vi "P116x2ch_WriteManual.vi"(5 "P116x2":T1, 7 "Enable(T)":bool=TRUE, 8 "error in (no error)":errorcluster, 9 "RateSP":T2, 10 "NuevoSP":T2, 11 "VISA Eurotherm":refnum<visa-resource-name>) -> (0 "error out":errorcluster, 1 "RateSP_out":T2, 2 "NuevoSP_out":T2)   [LabVIEW 2017]
uses:
  2xP116.ctl
  _P2024_P116x2w.ctl
  Address.ctl
  Eurotherm_2023_Module.ctl
  P2024 TB ICB GLOBALES.vi
panel:
  out "PV":T2
  out "WorkingSP":T2
  out "TargetSP":T2
  in  "Cancel":bool
  in  "Write":bool
  in  "Delay Time (s)":dbl=0.1
  # "Programando controladores P116"
  # "C/min"
  # "C"
  # "C"
  # "C"
  # "C"
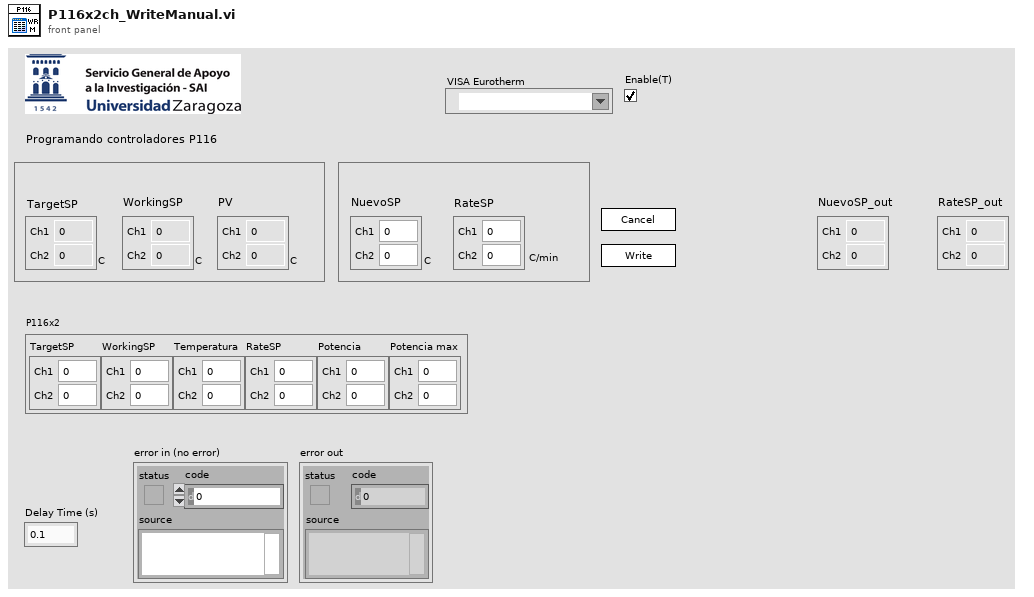
[diagram p1: front panel]
types:
  T1 = typedef "_P2024_P116x2w.ctl" = cluster{"TargetSP":T2, "WorkingSP":T2, "Temperatura":T2, "RateSP":T2, "Potencia":T2, "Potencia max":T2}
  T2 = typedef "2xP116.ctl" = cluster{"Ch1":dbl, "Ch2":dbl}
  T3 = typedef "_P2024 COMMS.ctl" = cluster{"Alicat":refnum<visa-resource-name>, "eAlic":bool, "Eurotherm":refnum<visa-resource-name>, "eEurot":bool, "Balanza":refnum<visa-resource-name>, "eBal":bool, "Valvula":refnum<visa-resource-name>, "eVal":bool}
  T4 = typedef "Eurotherm_2023_Module.ctl" = enum16{"Initialize", "Write setpoint", "Read data", "Write ramp rate", "Set constante proporcional", "Set constante integral", "Set constante diferencial", "Set ouput limit LOW", "Set ouput limit HIGH", "Shutdown"}
  T5 = typedef "Address.ctl" = enum16{"Add 1", "Add 2", "Add 3", "Add 4", "Add 5", "Add 6", "Add 10", "Add 11", "Add 12", "Add 13"}
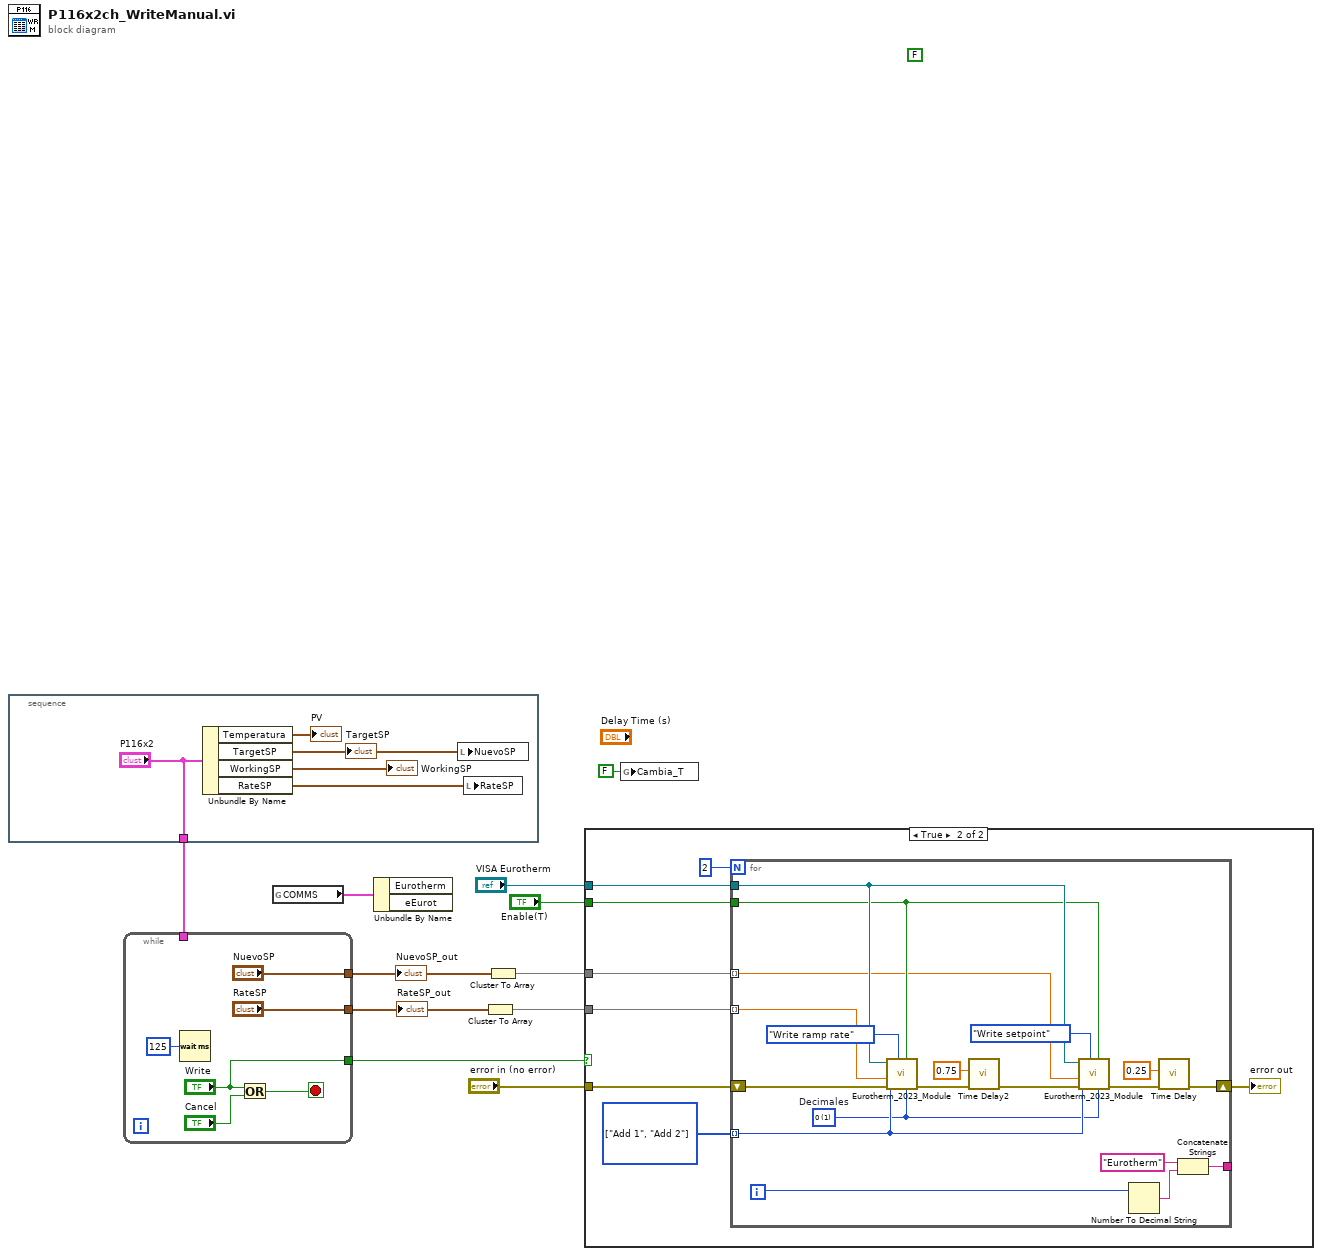
[diagram p0: block diagram]
diagram:
  (unwired) FALSE
  n1 = stacked-sequence {
    tunnel: ["P116x2"] -> w3
    frame #0 {
      n2 = Unbundle By Name("P116x2") -> ("Temperatura"=→"PV":T2, "TargetSP"=w14:T2, "WorkingSP"=→"WorkingSP":T2, "RateSP"=w12:T2)
      "TargetSP" <- w14
      n3 = local write "NuevoSP"(w14) -> ()
      n4 = local write "RateSP"(w12) -> ()
    }
  }
  n5 = while {
    tunnel: ["NuevoSP"] -> w1
    tunnel: ["RateSP"] -> w2
    tunnel: ["Write"] -> w6
    tunnel: w3 -> [_]
    stop <- w17 stop-if-true
    n6 = Wait (ms)(milliseconds to wait=u32 125) -> ()  [unwired: 1 out]
    n7 = Or(x="Write", y="Cancel") -> (x .or. y?=w17:bool)
  }
  "NuevoSP_out" <- w1
  "RateSP_out" <- w2
  n8 = global read "P2024 TB ICB GLOBALES.vi" "COMMS"() -> (w11:T3)
  n9 = Unbundle By Name(w11) -> ()  [unwired: 2 out]
  n10 = Cluster To Array(cluster=w2) -> (array=w7:dbl[])
  n11 = Cluster To Array(cluster=w1) -> (array=w8:dbl[])
  n12 = case shown="True" w6 {
    tunnel: "Enable(T)" -> [_ w29]
    tunnel: "error in (no error)" -> [_ w27]
    tunnel: w8 -> [_ w25]
    tunnel: w7 -> [_ w26]
    tunnel: "VISA Eurotherm" -> [_ w30]
    frame False {
    }
    frame True {
      w23 = T5[] [enum."Add 1", enum."Add 2"] items=["Add 1", "Add 2", "Add 3", "Add 4", "Add 5", "Add 6", "Add 10", "Add 11", "Add 12", "Add 13"]
      n13 = for {
        N: 2 -> [_]
        tunnel: w23 -> [w32] mode=indexing
        shift-right: [w37] -> w28
        shift-left: w27 -> [w44]
        tunnel: [w47] -> _
        tunnel: w25 -> [w39] mode=indexing
        tunnel: w26 -> [w40] mode=indexing
        tunnel: w30 -> [w43]
        tunnel: w29 -> [w42]
        i -> [w36]
        w31 = u16 1 items=["0"=1, "1"=10, "2"=100]  # Decimales
        n14 = call "Eurotherm_2023_Module.vi"("Decimales"=w31, "Eurotherm (T:Enable)"=w42, "Command"=Eurotherm_2023_Module."Write ramp rate", "error in (no error)"=w44, "Value"=w40, "Address"=w32, "VISA resource name"=w43) -> ("error out"=w34:errorcluster)  [unwired: 3 in, 1 out]
        n15 = call "Time Delay2"("error in (no error)"=w34, "Delay Time (s)"=0.75) -> ("error out"=w33:errorcluster)  [unwired: 9 in]
        n16 = call "Eurotherm_2023_Module.vi"("Decimales"=w31, "Eurotherm (T:Enable)"=w42, "Command"=Eurotherm_2023_Module."Write setpoint", "error in (no error)"=w33, "Value"=w39, "Address"=w32, "VISA resource name"=w43) -> ("error out"=w38:errorcluster)  [unwired: 3 in, 1 out]
        n17 = Number To Decimal String(number=w36) -> (decimal integer string=w48:string)  [unwired: 1 in]
        n18 = call "Time Delay"("error in (no error)"=w38, "Delay Time (s)"=0.25) -> ("error out"=w37:errorcluster)  [unwired: 9 in]
        n19 = Concatenate Strings("Eurotherm" ("error source (\" \")"), w48) -> (w47:string)
      }
      "error out" <- w28
    }
  }
  n20 = global write "P2024 TB ICB GLOBALES.vi" "Cambia_T"(FALSE ("ChangeT")) -> ()
